vi "Visualize Paths.vi"() -> ()   [LabVIEW 2022 SP3]
uses:
  FlexWorktable/FlexWorktable.lvclass
  Vec3d Class/Vec3d.lvclass
panel:
  out "new picture":picture
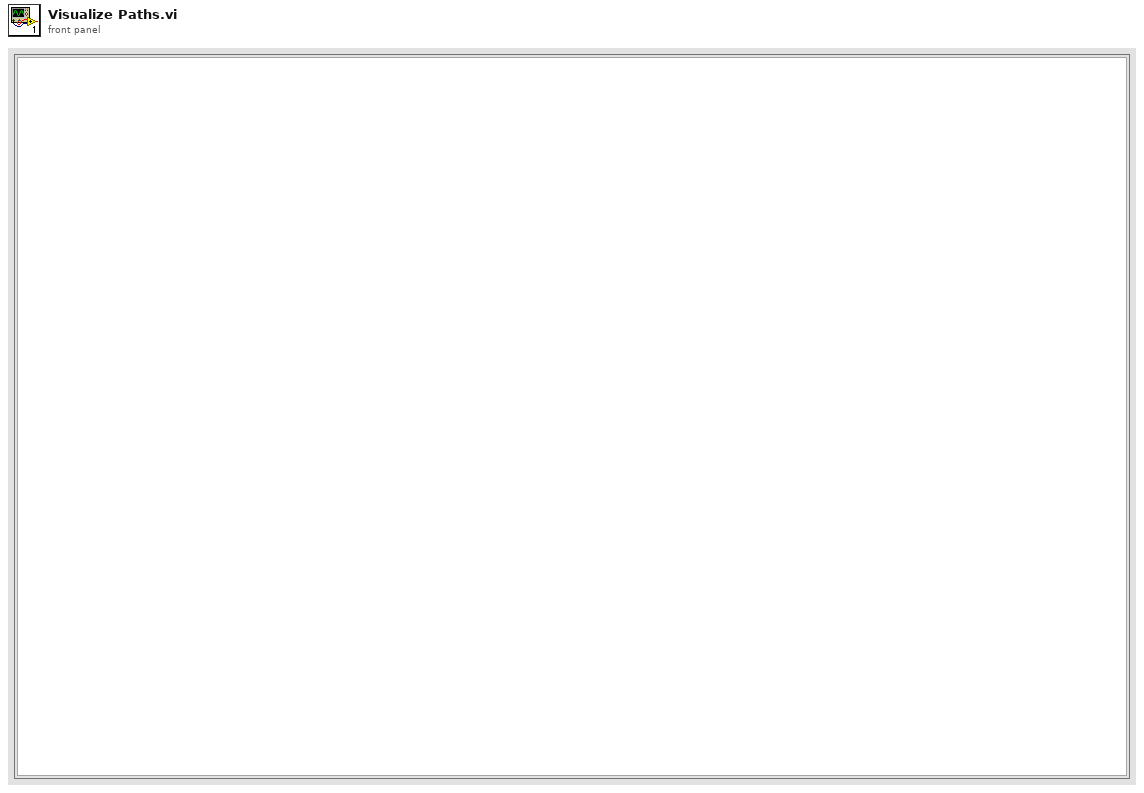
[diagram p1: front panel]
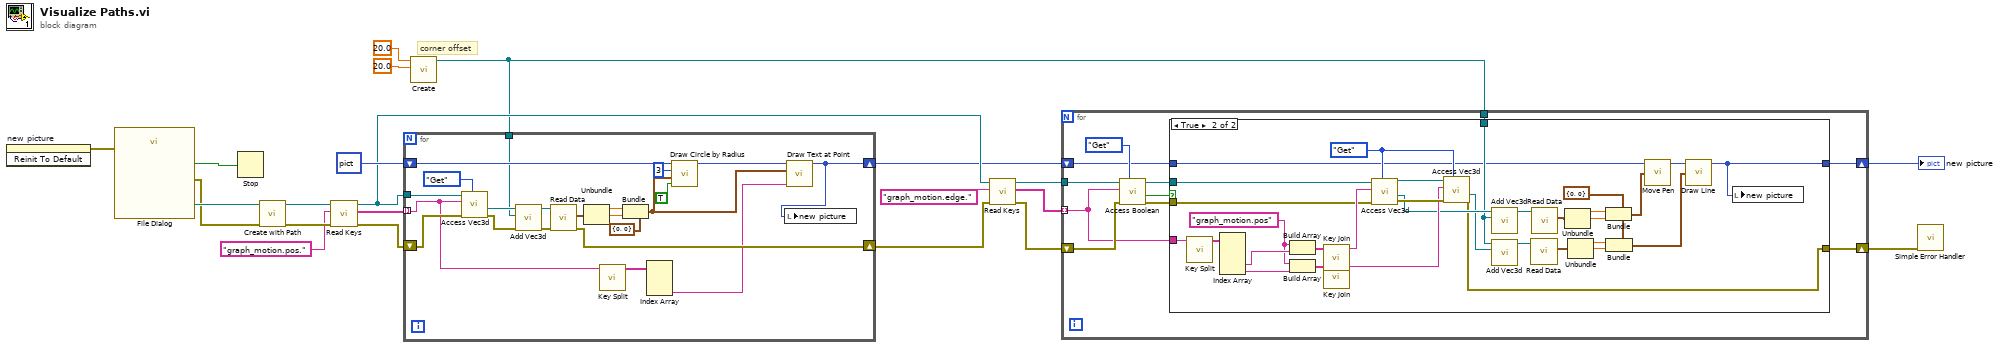
[diagram p0: block diagram]
diagram:
  # "corner offset"
  n1 = invoke on="new picture" class="Pict" method="Reinit To Default"() -> (error out=w2:errorcluster)  [unwired: 3 in, 2 out]
  n2 = call "File Dialog"("error in"=w2) -> ("selected path"=w5:path, "cancelled"=w4:bool, "error out"=w3:errorcluster)  [unwired: 11 in, 1 out]
  n3 = Stop(stop? (T)=w4) -> ()
  n4 = call "Create with Path.vi"("error in (no error)"=w3, "flex_config path"=w5) -> ("error out"=w21:errorcluster, "FlexWorktable out"=w22:refnum<class "FlexWorktable.lvclass">)  [unwired: 8 in]
  n5 = call-dynamic "Read Keys.vi"("error in (no error)"=w21, "Selector"="graph_motion.pos.", "FlexWorktable in"=w22) -> ("error out"=w17:errorcluster, "Keys"=w19:string[], "FlexWorktable out"=w16:refnum<class "FlexWorktable.lvclass">)  [unwired: 6 in]
  n6 = call "Create.vi"("Y"=20.0, "X"=20.0) -> ("Vec3d Class out"=w6:refnum<class "Vec3d.lvclass">)  [unwired: 8 in, 1 out]
  n7 = for {
    tunnel: w19 -> [w26] mode=indexing
    shift-right: [w23] -> w15
    shift-left: picture data[5B] ("picture") -> [w39]
    tunnel: w16 -> [w44]
    shift-right: [w40] -> w13
    shift-left: w17 -> [w43]
    tunnel: w6 -> [w29]
    n8 = call-dynamic "Access Vec3d.vi"("Get/Set"=enum16{"Get", "Set"}."Get", "error in (no error)"=w43, "Key"=w26, "FlexWorktable in"=w44) -> ("error out"=w31:errorcluster, "Value out"=w33:refnum<class "Vec3d.lvclass">)  [unwired: 5 in, 1 out]
    n9 = call-dynamic "Add Vec3d.vi"("error in (no error)"=w31, 10:"Vec3d Class in"=w29, 11:"Vec3d Class in"=w33) -> ("error out"=w30:errorcluster, "Vec3d Class out"=w32:refnum<class "Vec3d.lvclass">)  [unwired: 7 in]
    n10 = call-dynamic "Read Data.vi"("error in (no error)"=w30, "Vec3d Class in"=w32) -> ("error out"=w40:errorcluster, "Data"=w41:cluster{"X":dbl, "Y":dbl, "Z":dbl})  [unwired: 7 in, 1 out]
    n11 = Unbundle(w41) -> ("X"=w35:dbl, "Y"=w34:dbl)  [unwired: 1 out]
    n12 = call "Key Split.vi"("Key"=w26) -> ("Key Elements"=w25:string[])  [unwired: 10 in]
    n13 = Bundle(cluster=cluster{"horizontal":i16, "vertical":i16} {"horizontal"=0, "vertical"=0} ("pixel center"), "horizontal"=w35, "vertical"=w34) -> (w27:cluster{"horizontal":i16, "vertical":i16})
    n14 = Index Array(array=w25) -> (element #3=w24:string)  [unwired: 3 in, 2 out]
    n15 = call <vilib>:"Draw Circle by Radius.vi"("fill?(F)"=TRUE, "pixel center"=w27, "radius"=i16 3, "picture"=w39) -> ("new picture"=w28:picture)  [unwired: 7 in]
    n16 = call <vilib>:"Draw Text at Point.vi"("text"=w24, "origin"=w27, "picture"=w28) -> ("new picture"=w23:picture)  [unwired: 7 in, 1 out]
    n17 = local write "new picture"(w23) -> ()
  }
  n18 = call-dynamic "Read Keys.vi"("error in (no error)"=w13, "Selector"="graph_motion.edge.", "FlexWorktable in"=w16) -> ("error out"=w12:errorcluster, "Keys"=w10:string[], "FlexWorktable out"=w11:refnum<class "FlexWorktable.lvclass">)  [unwired: 6 in]
  n19 = for {
    shift-right: [w46] -> w9
    shift-left: w15 -> [w47]
    shift-right: [w48] -> w1
    shift-left: w12 -> [w54]
    tunnel: w11 -> [w55]
    tunnel: w10 -> [w53] mode=indexing
    tunnel: w6 -> [w45]
    n20 = call-dynamic "Access Boolean.vi"("Get/Set"=enum16{"Get", "Set"}."Get", "error in (no error)"=w54, "Key"=w53, "FlexWorktable in"=w55) -> ("error out"=w49:errorcluster, "Value out"=w51:bool, "FlexWorktable out"=w50:refnum<class "FlexWorktable.lvclass">)  [unwired: 5 in]
    n21 = case shown="True" w51 {
      tunnel: w53 -> [_ w89]
      tunnel: w50 -> [_ w87]
      tunnel: w49 -> [w57 w80]
      tunnel: [w57 w59] -> w48
      tunnel: w47 -> [w56 w72]
      tunnel: [w56 w58] -> w46
      tunnel: w45 -> [_ w73]
      frame False {
      }
      frame True {
        w62 = cluster{"x":i16, "y":i16} {"x"=0, "y"=0} ("new position")
        w83 = "graph_motion.pos"
        w79 = enum16{"Get", "Set"}."Get" ("Get/Set")
        n22 = call "Key Split.vi"("Key"=w89) -> ("Key Elements"=w88:string[])  [unwired: 10 in]
        n23 = Index Array(array=w88) -> (element #3=w85:string, element #4=w82:string)  [unwired: 4 in, 2 out]
        n24 = Build Array(w83, w85) -> (w86:string[])
        n25 = Build Array(w83, w82) -> (w84:string[])
        n26 = call "Key Join.vi"("Key Elements"=w86) -> ("Key"=w81:string)  [unwired: 10 in]
        n27 = call "Key Join.vi"("Key Elements"=w84) -> ("Key"=w76:string)  [unwired: 10 in]
        n28 = call-dynamic "Access Vec3d.vi"("Get/Set"=w79, "error in (no error)"=w80, "Key"=w81, "FlexWorktable in"=w87) -> ("error out"=w78:errorcluster, "Value out"=w75:refnum<class "Vec3d.lvclass">, "FlexWorktable out"=w77:refnum<class "FlexWorktable.lvclass">)  [unwired: 5 in]
        n29 = call-dynamic "Access Vec3d.vi"("Get/Set"=w79, "error in (no error)"=w78, "Key"=w76, "FlexWorktable in"=w77) -> ("error out"=w59:errorcluster, "Value out"=w74:refnum<class "Vec3d.lvclass">)  [unwired: 5 in, 1 out]
        n30 = call-dynamic "Add Vec3d.vi"(10:"Vec3d Class in"=w73, 11:"Vec3d Class in"=w75) -> ("Vec3d Class out"=w70:refnum<class "Vec3d.lvclass">)  [unwired: 8 in, 1 out]
        n31 = call-dynamic "Add Vec3d.vi"(10:"Vec3d Class in"=w74, 11:"Vec3d Class in"=w73) -> ("Vec3d Class out"=w69:refnum<class "Vec3d.lvclass">)  [unwired: 8 in, 1 out]
        n32 = call-dynamic "Read Data.vi"("Vec3d Class in"=w69) -> ("Data"=w67:cluster{"X":dbl, "Y":dbl, "Z":dbl})  [unwired: 8 in, 2 out]
        n33 = call-dynamic "Read Data.vi"("Vec3d Class in"=w70) -> ("Data"=w68:cluster{"X":dbl, "Y":dbl, "Z":dbl})  [unwired: 8 in, 2 out]
        n34 = Unbundle(w68) -> ("X"=w66:dbl, "Y"=w65:dbl)  [unwired: 1 out]
        n35 = Unbundle(w67) -> ("X"=w63:dbl, "Y"=w61:dbl)  [unwired: 1 out]
        n36 = Bundle(cluster=w62, "x"=w66, "y"=w65) -> (w64:cluster{"x":i16, "y":i16})
        n37 = Bundle(cluster=w62, "x"=w63, "y"=w61) -> (w60:cluster{"x":i16, "y":i16})
        n38 = call <vilib>:"Move Pen.vi"("new position"=w64, "picture"=w72) -> ("new picture"=w71:picture)  [unwired: 3 in]
        n39 = call <vilib>:"Draw Line.vi"("picture"=w71, "end point"=w60) -> ("new picture"=w58:picture)  [unwired: 7 in]
        n40 = local write "new picture"(w58) -> ()
      }
    }
  }
  "new picture" <- w9
  n41 = call <vilib>:"Simple Error Handler.vi"("error in (no error)"=w1) -> ()  [unwired: 4 in, 5 out]
